vi "Get Color Frame.vi"(8 "error in (no error)":errorcluster, 11 "Kinect Session in":refnum<class "Kinect Session.lvclass">) -> (0 "error out":errorcluster, 2 "Color Frame":T1(plugin-control), 3 "Kinect Session out":refnum<class "Kinect Session.lvclass">)   [LabVIEW 2014, in "Kinect Library.lvlib"]
doc: "This VI will retrieve the latest image. If this function is called too frequently, it can return an error. If the function is called too sparsely, nothing bad will happen."
uses:
  Kinect Library.lvlib
  Kinect Session Class/Kinect Session.lvclass
  Microsoft.Kinect
  <vilib>/vision/NI_Vision_Development_Module.lvlib
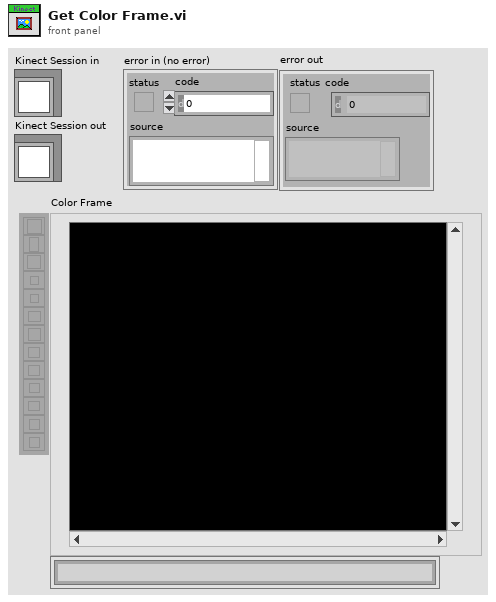
[diagram p1: front panel]
types:
  T1 = typedef "IMAQ Image.ctl" = refnum<image>
  T2 = cluster{"FramePixelDataLength":i32, "FrameWidth":i32, "FrameHeight":i32}
  T3 = cluster{"status":bool, "code":bool, "source":bool}
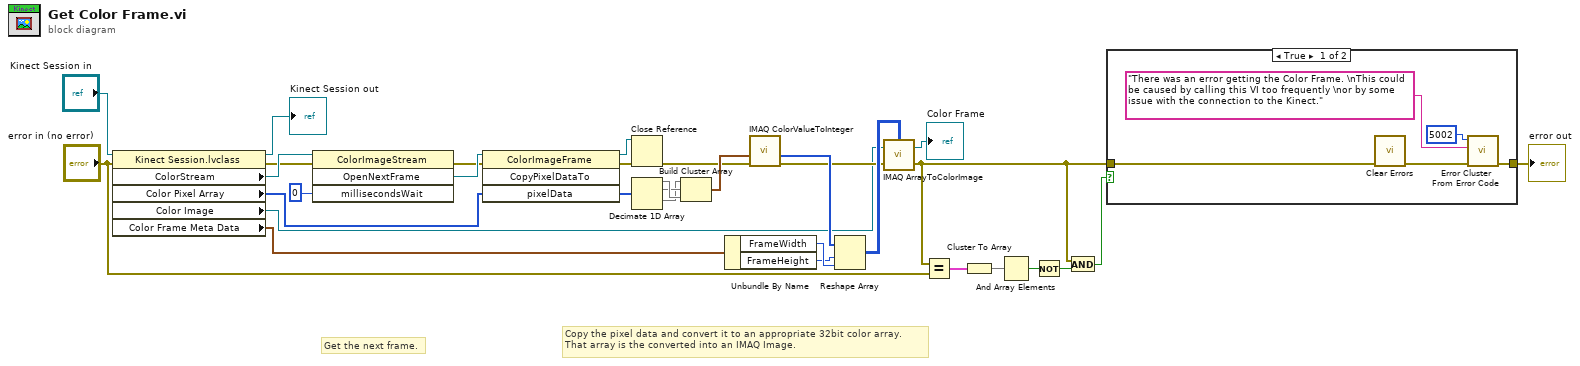
[diagram p0: block diagram]
diagram:
  # "Copy the pixel data and convert it to an appropriate 32bit color array.\nThat array is the converted into an IMAQ Image."
  # "Get the next frame."
  n1 = property class="Kinect Session.lvclass"(reference="Kinect Session in", error in="error in (no error)") -> (reference out=→"Kinect Session out":refnum<class "Kinect Session.lvclass">, error out=w9:errorcluster, "ColorStream"=w17:refnum<k24>, "Color Pixel Array"=w15:u8[], "Color Image"=w14:T1, "Color Frame Meta Data"=w13:T2)
  n2 = invoke class="ColorImageStream" method="OpenNextFrame"(reference=w17, error in=w9, "millisecondsWait"=0) -> (error out=w27:errorcluster, "OpenNextFrame"=w32:refnum<k24>)  [unwired: 1 in, 2 out]
  n3 = invoke class="ColorImageFrame" method="CopyPixelDataTo"(reference=w32, error in=w27, "pixelData"=w15) -> (reference out=w22:refnum<k24>, error out=w21:errorcluster, "pixelData"=w31:u8[])  [unwired: 1 in, 1 out]
  n4 = Close Reference(reference=w22, error in (no error)=w21) -> (error out=w19:errorcluster)
  n5 = Decimate 1D Array(w31) -> (w26:u8[], w25:u8[], w24:u8[])  [unwired: 1 out]
  n6 = Build Cluster Array(w24, w25, w26) -> (w23:cluster{u8, u8, u8}[])
  n7 = Unbundle By Name(w13) -> ("FrameWidth"=w12:i32, "FrameHeight"=w11:i32)
  n8 = call "IMAQ ColorValueToInteger"("error in (no error)"=w19, "1D Color value array"=w23) -> ("1D U32 array"=w30:u32[], "error out"=w20:errorcluster)  [unwired: 3 in, 2 out]
  n9 = Reshape Array(w30, w11, w12) -> (w29:u32[][])
  n10 = call "IMAQ ArrayToColorImage"("Image Pixels (U32)"=w29, "Image"=w14, "error in (no error)"=w20) -> ("Image Out"=→"Color Frame":T1, "error out"=w4:errorcluster)  [unwired: 2 in]
  n11 = Equal?(x=w4, y="error in (no error)") -> (x = y?=w8:T3)
  n12 = Cluster To Array(cluster=w8) -> (array=w7:bool[])
  n13 = And Array Elements(Boolean array=w7) -> (logical AND=w3:bool)
  n14 = Not(x=w3) -> (.not. x?=w6:bool)
  n15 = And(x=w4, y=w6) -> (x .and. y?=w2:bool)
  n16 = case shown="True" w2 {
    tunnel: [w37 w38] -> w1
    tunnel: w4 -> [w34 w38]
    frame True {
      n17 = call <vilib>:"Clear Errors.vi"("error in (no error)"=w34) -> ("error out"=w33:errorcluster)  [unwired: 5 in, 1 out]
      n18 = call <vilib>:"Error Cluster From Error Code.vi"("error in (no error)"=w33, "error message (\"\")"="There was an error getting the Color Frame. \nThis could be caused by calling this VI too frequently \nor by some issue with the connection to the Kinect." ("error message (\"\")"), "error code (0)"=5002) -> ("error out"=w37:errorcluster)  [unwired: 6 in]
    }
    frame False {
    }
  }
  "error out" <- w1
